vi "NewContact.vi"(7 "LabVIEW Web Service Request":refnum<class "Web Request.lvclass">) -> ()   [LabVIEW 2014]
doc: "This HTTP Method VI shows the new contact form, which is submitted to the EditContact method."
uses:
  <vilib>/wsapi/Web Request.lvclass
  <vilib>/wsapi/class/subVIs/Set String ESP Variable.vi
panel:
  # "Because this is an HTTP Method VI, LabVIEW Web Service Request is populated automatically."
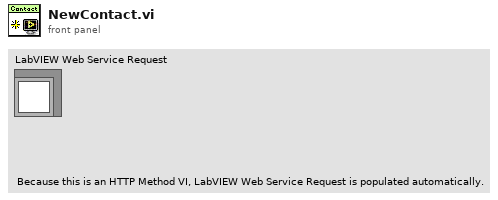
[diagram p1: front panel]
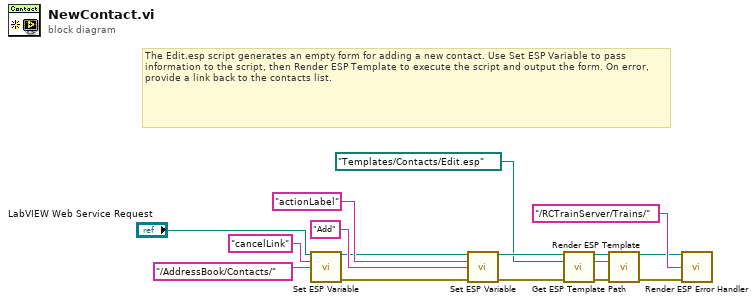
[diagram p0: block diagram]
diagram:
  # "The Edit.esp script generates an empty form for adding a new contact. Use Set ESP Variable to pass information to the script, then Render ESP Template to execute the script and output the form. On error, provide a link back to the contacts list."
  n1 = call-poly <vilib>:"Set ESP Variable.vi"("LabVIEW Web Service Request"="LabVIEW Web Service Request", "key"="cancelLink", "value"="/AddressBook/Contacts/") -> ("LabVIEW Web Service Request out"=w12:refnum<class "Web Request.lvclass">, "error out"=w10:errorcluster)  [unwired: 11 in]
  n2 = call-poly <vilib>:"Set ESP Variable.vi"("LabVIEW Web Service Request"=w12, "key"="actionLabel", "value"="Add", "error in (no error)"=w10) -> ("LabVIEW Web Service Request out"=w9:refnum<class "Web Request.lvclass">, "error out"=w8:errorcluster)  [unwired: 10 in]
  n3 = call "Get ESP Template Path.vi"("LabVIEW Web Service Request"=w9, "Relative Template Path"=path "Templates/Contacts/Edit.esp", "error in (no error)"=w8) -> ("LabVIEW Web Service Request out"=w6:refnum<class "Web Request.lvclass">, "Template Name"=w5:string, "error out"=w7:errorcluster)  [unwired: 10 in]
  n4 = call <vilib>:"Render ESP Template.vi"("LabVIEW Web Service Request"=w6, "espName"=w5, "error in (no error)"=w7) -> ("LabVIEW Web Service Request out"=w1:refnum<class "Web Request.lvclass">, "error out"=w3:errorcluster)  [unwired: 11 in]
  n5 = call "Render ESP Error Handler.vi"("LabVIEW Web Service Request"=w1, "Link"="/RCTrainServer/Trains/", "error in (no error)"=w3) -> ()  [unwired: 11 in, 2 out]
